vi "U6 Single AIN Example mod.vi"(8 "error in":errorcluster, 9 "AIN Range":u16(ring) items=["LJ_rgBIP10V", "LJ_rgBIP1V", "LJ_rgBIPP1V", "LJ_rgBIPP01V"], 10 "Negative Channel #":i32=199, 11 "Positive Channel #":i32) -> (0 "error out":errorcluster, 2 "Value Read":dbl format="%.9f")   [LabVIEW 2021]
panel:
  in  "Binary":bool
  in  "SettlingFactor":i32
  in  "Resolution":i32
  in  "FirstFound":bool=TRUE
  in  "Address":string="1"
  out "Error Message":string
  # "Configures and reads 1 analog input."
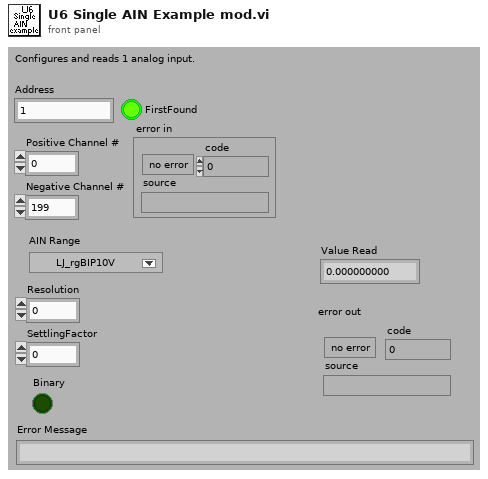
[diagram p1: front panel]
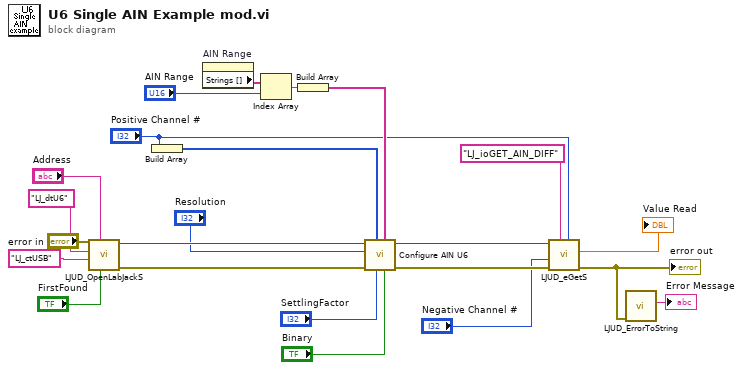
[diagram p0: block diagram]
diagram:
  n1 = call <vilib>:"LJUD_OpenLabJackS.vi"("FirstFound"="FirstFound", "Address"="Address", "error in"="error in", "ConnectionType"="LJ_ctUSB", "DeviceType"="LJ_dtU6") -> ("error out"=w12:errorcluster, "Handle"=w13:i32)  [unwired: 4 in, 1 out]
  n2 = Build Array("Positive Channel #") -> (w9:i32[])
  n3 = property on="AIN Range" class="Ring (strict)"() -> ("Strings []"=w11:string[])  [unwired: 2 in, 2 out]
  n4 = Index Array(array=w11, index="AIN Range") -> (element=w8:string)
  n5 = Build Array(w8) -> (w7:string[])
  n6 = call <vilib>:"Configure AIN U6.vi"("Binary"="Binary", "Ranges"=w7, "SettlingFactor"="SettlingFactor", "Positive Channels"=w9, "error in"=w12, "Resolution"="Resolution", "Handle In"=w13) -> ("error out"=w15:errorcluster, "Handle Out"=w14:i32)  [unwired: 3 in]
  n7 = call <vilib>:"LJUD_eGetS.vi"("Channel"="Positive Channel #", "IOType"="LJ_ioGET_AIN_DIFF", "error in"=w15, "x1"="Negative Channel #", "Handle In"=w14) -> ("error out"=w20:errorcluster, "Value Read"=→"Value Read":dbl)  [unwired: 4 in, 1 out]
  "error out" <- w20
  n8 = call <vilib>:"LJUD_ErrorToString.vi"("error in"=w20) -> ("String"=→"Error Message":string)  [unwired: 10 in]
